vi "SetSize.vi"(8 "error in (no error)":errorcluster, 10 "Size":u32, 11 "ArbitraryFunction in":refnum<class "ArbitraryFunction.lvclass">) -> (0 "error out":errorcluster, 3 "ArbitraryFunction out":refnum<class "ArbitraryFunction.lvclass">)   [LabVIEW 2018, in "Functions.lvlib" / "ArbitraryFunction.lvclass"]
uses:
  ArbitraryFunction.lvclass
  ArbitraryFunction.lvclass/ArbitraryFunction.ctl
  Accessors/Read Arbs.vi
  Accessors/Write Arbs.vi
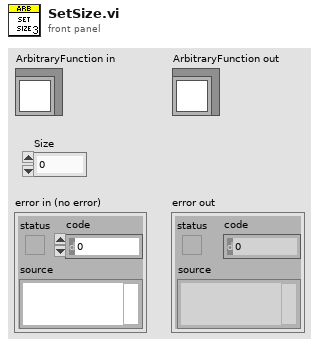
[diagram p1: front panel]
types:
  T1 = typedef "Functions.lvlib/ArbitraryFunction.lvclass/Arbitrary.ctl" = cluster{"Handle":string, "Size":i32, "Gain":dbl, "Offset":dbl, "Waveform":waveform(dbl)}
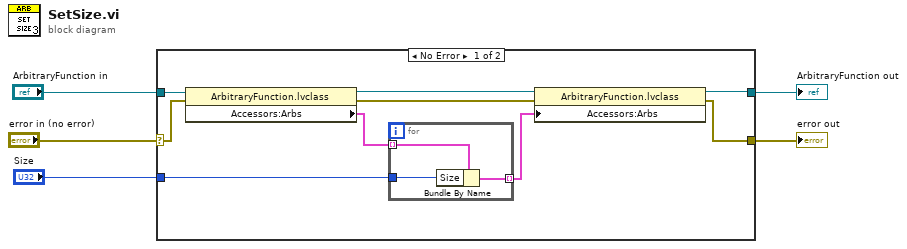
[diagram p0: block diagram]
diagram:
  n1 = case shown="No Error" "error in (no error)" {
    selector: "error in (no error)" -> [w13 w19]
    tunnel: [w6 w19] -> w5
    tunnel: "ArbitraryFunction in" -> [w14 w18]
    tunnel: [w11 w18] -> w3
    tunnel: "Size" -> [w9 _]
    frame No Error {
      n2 = property class="ArbitraryFunction.lvclass"(reference=w14, error in=w13) -> (reference out=w12:refnum<class "ArbitraryFunction.lvclass">, error out=w7:errorcluster, "Accessors:Arbs"=w10:T1[])
      n3 = for {
        tunnel: w10 -> [w17] mode=indexing
        tunnel: w9 -> [w16]
        tunnel: [w15] -> w8 mode=indexing
        n4 = Bundle By Name(cluster=w17, "Size"=w16) -> (w15:T1)
      }
      n5 = property class="ArbitraryFunction.lvclass"(reference=w12, error in=w7, "Accessors:Arbs"=w8) -> (reference out=w11:refnum<class "ArbitraryFunction.lvclass">, error out=w6:errorcluster)
    }
    frame Error {
    }
  }
  "error out" <- w5
  "ArbitraryFunction out" <- w3
